vi "Header Value.vi"(8 "error in (no error)":errorcluster, 10 "Header":string, 11 "Response in":refnum<class "Response.lvclass">) -> (0 "error out":errorcluster, 1 "Exists":bool, 2 "Value":string, 3 "Response out":refnum<class "Response.lvclass">)   [LabVIEW 2020, in "HTTP Utils.lvlib" / "Response.lvclass"]
uses:
  Response.lvclass
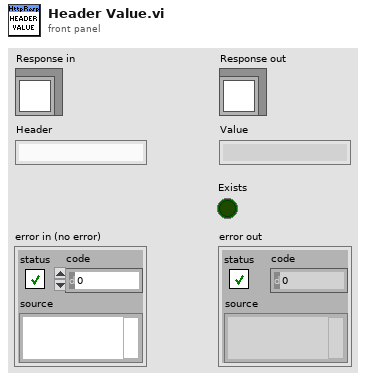
[diagram p1: front panel]
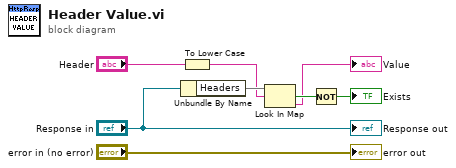
[diagram p0: block diagram]
diagram:
  n1 = Unbundle By Name("Response in") -> ("Headers"=w7:map{string, string})
  n2 = To Lower Case(string="Header") -> (all lower case string=w5:string)
  n3 = Look In Map(map=w7, key=w5) -> (key not found?=w6:bool, value=→"Value":string)  [unwired: 1 in]
  n4 = Not(x=w6) -> (.not. x?=→"Exists":bool)
  "error out" <- "error in (no error)"
  "Response out" <- "Response in"
